vi "Kinesis - KBD101 - Set Trigger Parameters.vi"() -> ()   [LabVIEW 2012]
uses:
  U:/Kinesis LabVIEW Website Examples/Thorlabs.MotionControl.Controls.dll
  Thorlabs.MotionControl.Controls.dll
  U:/Kinesis LabVIEW Website Examples/Thorlabs.MotionControl.KCube.BrushlessMotorCLI.dll
  Thorlabs.MotionControl.KCube.BrushlessMotorCLI.dll
  U:/Kinesis LabVIEW Website Examples/Thorlabs.MotionControl.GenericMotorCLI.dll
  Thorlabs.MotionControl.GenericMotorCLI.dll
panel:
  in  "?":bool
  in  "stop":bool
  in  "SerialNumber":string
  in  "Trigger2Polarity":i32(ring)=1 items=["TriggerHigh"=1, "TriggerLow"=2]
  in  "Trigger2Mode":i32(ring) items=["Disabled"=0, "TrigIN_GPI"=1, "TrigIN_RelativeMove"=2, "TrigIN_AbsoluteMove"=3, "TrigIN_KCubeTriggerParams"=4, "TrigOUT_GPO"=10, "TrigOUT_InMotion"=11, "TrigOUT_AtMaxVelocity"=12, "TrigOUT_AtPositionFwd"=13, "TrigOUT_AtPositionRev"=14, "TrigOUT_AtPositionBoth"=15, "TrigOut_AtFwdLimit"=16, "TrigOut_AtBwdLimit"=17, "TrigOut_AtLimit"=18]
  in  "Trigger1Polarity":i32(ring)=1 items=["TriggerHigh"=1, "TriggerLow"=2]
  out "Trigger2Polarity":i32(ring)=1 items=["TriggerHigh"=1, "TriggerLow"=2]
  out "Trigger2Mode":i32(ring) items=["Disabled"=0, "TrigIN_GPI"=1, "TrigIN_RelativeMove"=2, "TrigIN_AbsoluteMove"=3, "TrigIN_KCubeTriggerParams"=4, "TrigOUT_GPO"=10, "TrigOUT_InMotion"=11, "TrigOUT_AtMaxVelocity"=12, "TrigOUT_AtPositionFwd"=13, "TrigOUT_AtPositionRev"=14, "TrigOUT_AtPositionBoth"=15, "TrigOut_AtFwdLimit"=16, "TrigOut_AtBwdLimit"=17, "TrigOut_AtLimit"=18]
  out "Trigger1Polarity":i32(ring)=1 items=["TriggerHigh"=1, "TriggerLow"=2]
  in  "Trigger1Mode":i32(ring) items=["Disabled"=0, "TrigIN_GPI"=1, "TrigIN_RelativeMove"=2, "TrigIN_AbsoluteMove"=3, "TrigIN_KCubeTriggerParams"=4, "TrigOUT_GPO"=10, "TrigOUT_InMotion"=11, "TrigOUT_AtMaxVelocity"=12, "TrigOUT_AtPositionFwd"=13, "TrigOUT_AtPositionRev"=14, "TrigOUT_AtPositionBoth"=15, "TrigOut_AtFwdLimit"=16, "TrigOut_AtBwdLimit"=17, "TrigOut_AtLimit"=18]
  out "Trigger1Mode":i32(ring) items=["Disabled"=0, "TrigIN_GPI"=1, "TrigIN_RelativeMove"=2, "TrigIN_AbsoluteMove"=3, "TrigIN_KCubeTriggerParams"=4, "TrigOUT_GPO"=10, "TrigOUT_InMotion"=11, "TrigOUT_AtMaxVelocity"=12, "TrigOUT_AtPositionFwd"=13, "TrigOUT_AtPositionRev"=14, "TrigOUT_AtPositionBoth"=15, "TrigOut_AtFwdLimit"=16, "TrigOut_AtBwdLimit"=17, "TrigOut_AtLimit"=18]
  in  "TriggerStartPositionRev":dbl
  in  "TriggerStartPositionFwd":dbl
  in  "TriggerPulseWidth":i32
  in  "TriggerIntervalRev":dbl
  in  "TriggerIntervalFwd":dbl
  in  "TriggerCountRev":i32
  in  "CycleCount":i32
  in  "TriggerCountFwd":i32
  out "TriggerStartPositionRev":dbl
  out "TriggerStartPositionFwd":dbl
  out "TriggerPulseWidth":i32
  out "TriggerIntervalRev":dbl
  out "TriggerIntervalFwd":dbl
  out "TriggerCountRev":i32
  out "TriggerCountFwd":i32
  out "CycleCount":i32
  in  "KCubeBrushlessControl":refnum<k24>(container)
  # "Notes:"
  # "- Ensure that the appropriate .DLLs are copied into your Project Folder. Check that the correct bit type are used depending on your version of LabVIEW\ni.e. 32-bit or 64-bit.\n\n\n\n\n\n\n\n\n\n\n\n\n\n\n- Open the example VI through the LabVIEW Project Explorer to correctly load the User Interface from Thorlabs.MotionControl.Controls.dll."
  # "Thorlabs Hardware: KBD101 - K-Cube Brushless DC Servo Motor Controller\nhttps://www.thorlabs.com/thorproduct.cfm?partnumber=KBD101\n\nDescription: This VI will enable you to explore the Trigger Parameters available to all Thorlabs K-Cube devices. In this case, the VI will accept a KBD101 controller specifically.\n\nInstructions: \n1) Connect your KBD101 device to your PC & power the device, ensuring your stage/actutator is connected. For full device setup, the device product manual can be found on our website here. - https://www.thorlabs.com/thorproduct.cfm?partnumber=KBD101\n2) Enter the device serial number below.\n3) Click 'Run' in the LabVIEW Toolbar.\n4) Enter parameters for Trigger Settings in the controls below. Further details of these parameters are outlined in the KBD101 product manual, as well as the Kinesis .NET API.\n5) Click 'SET TRIG PARAMETERS' to set the Trigger Parameters. The program will poll for clicks every 500ms.\n6) Click 'END PROGRAM' to end the VI."
  # "Example Image of .NET Controller - VI opened via Project Explorer/ not opened via Project Explorer"
  # "VI Not Opened via Project Explorer"
  # "VI Opened via Project Explorer"
  # "- To explore the range of methods available, please visit the .NET API, included with your Kinesis software.\n\n- For tips on building your own VIs with Thorlabs Motion Control Hardware, please see our LabVIEW Guide here.\nhttps://www.thorlabs.com/newgrouppage9.cfm?objectgroup_id=10285"
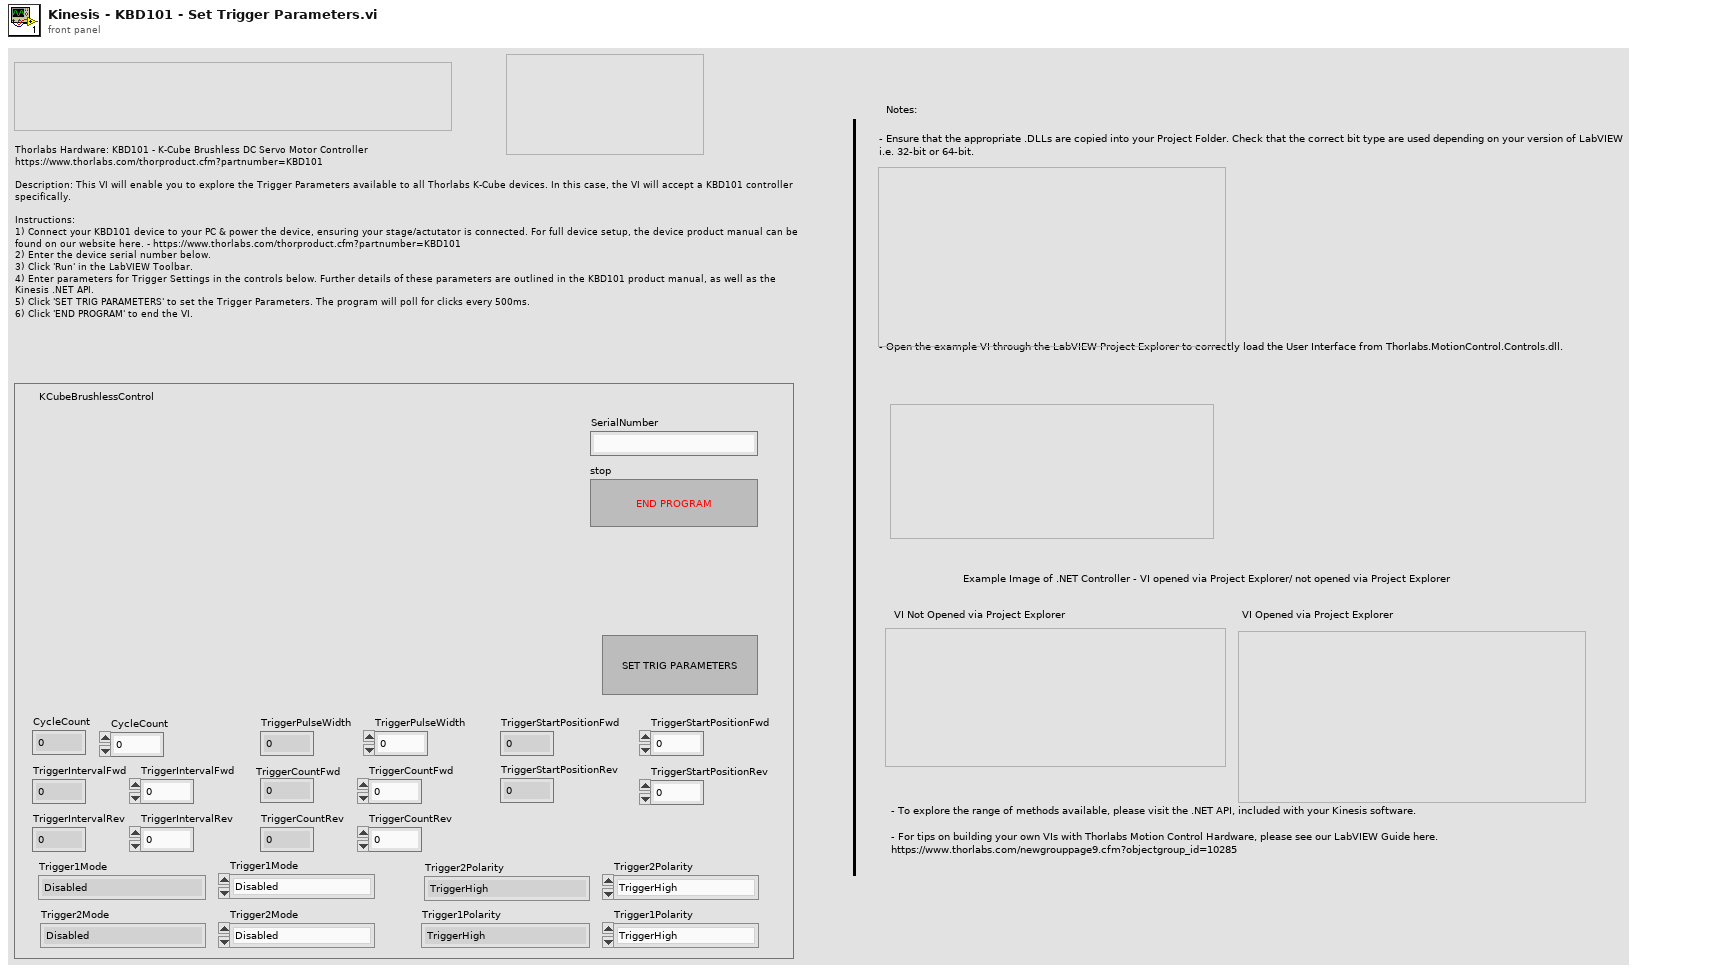
[diagram p1: front panel]
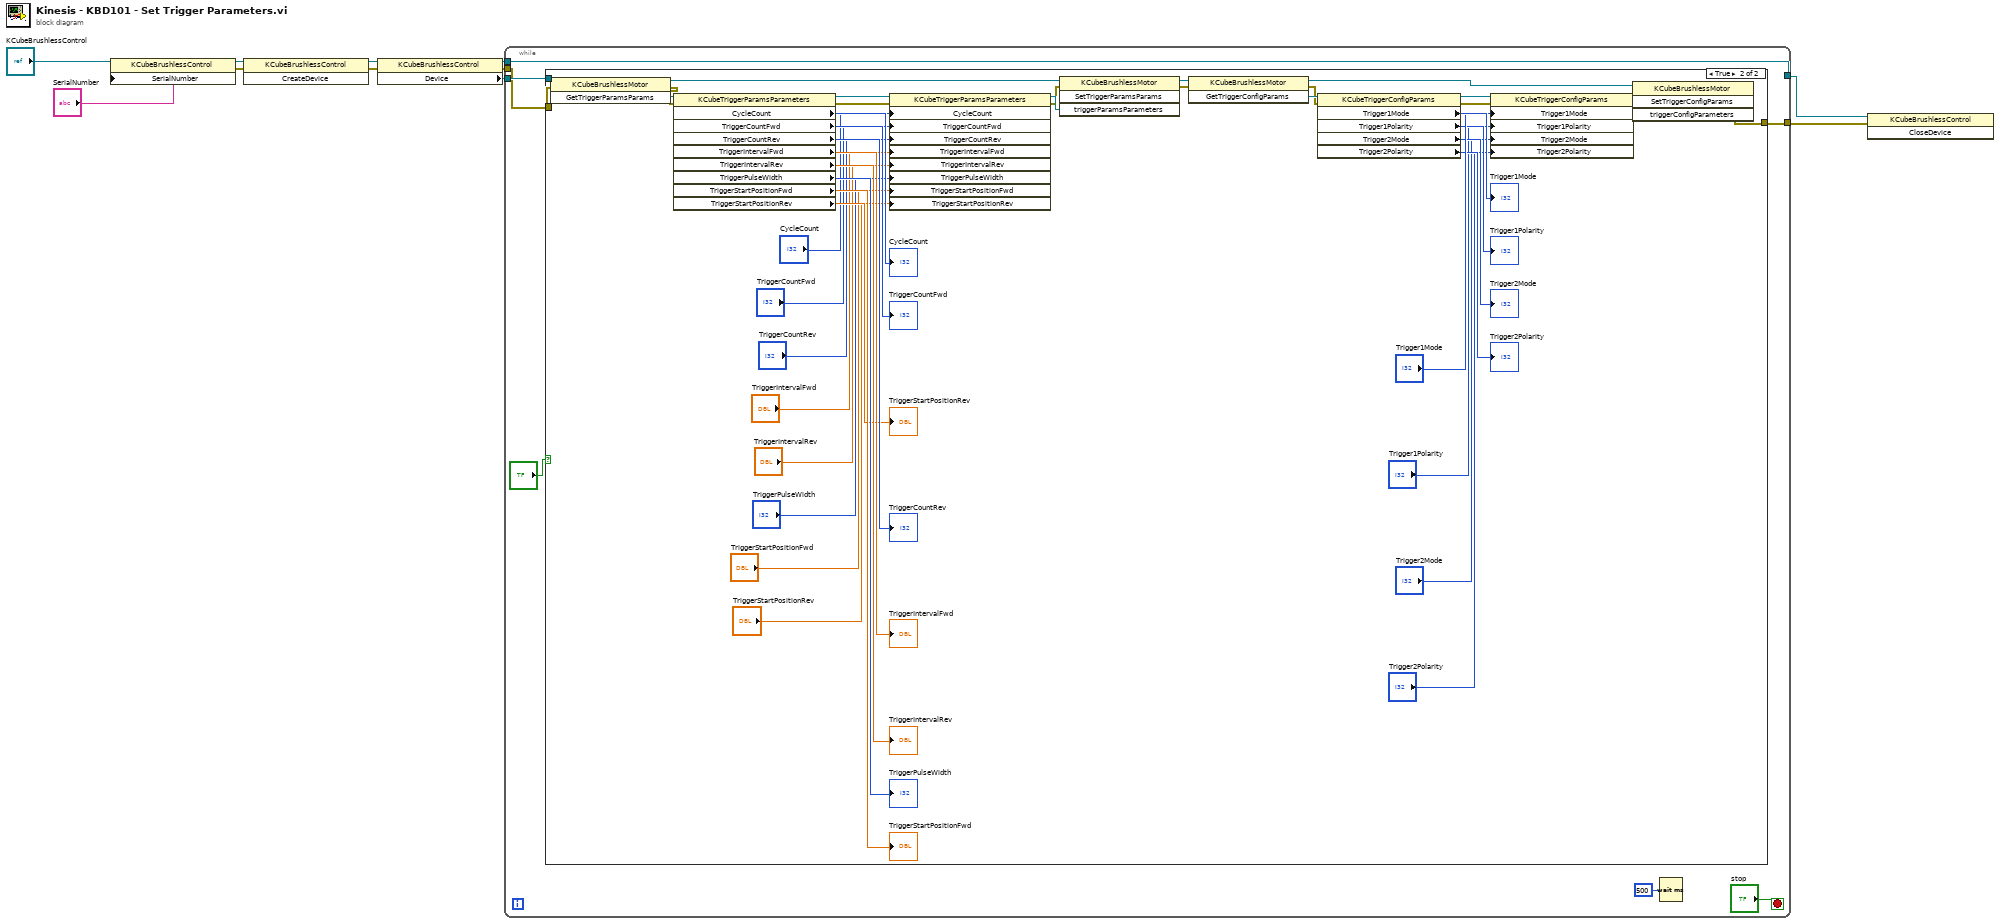
[diagram p0: block diagram]
diagram:
  n1 = property class="KCubeBrushlessControl"(reference="KCubeBrushlessControl", "SerialNumber"="SerialNumber") -> (reference out=w10:refnum<k24>, error out=w4:errorcluster)  [unwired: 1 in]
  n2 = invoke class="KCubeBrushlessControl" method="CreateDevice"(reference=w10, error in=w4) -> (reference out=w9:refnum<k24>, error out=w3:errorcluster)  [unwired: 1 in, 1 out]
  n3 = property class="KCubeBrushlessControl"(reference=w9, error in=w3) -> (reference out=w6:refnum<k24>, error out=w2:errorcluster, "Device"=w8:refnum<k24>)
  n4 = while {
    tunnel: w8 -> [w18]
    tunnel: [w16] -> w5
    tunnel: w6 -> [w16]
    tunnel: w2 -> [w15]
    tunnel: [w14] -> w1
    stop <- "stop" stop-if-true
    n5 = case shown="True" "?" {
      tunnel: w18 -> [_ w62]
      tunnel: w15 -> [w19 w28]
      tunnel: [w19 w20] -> w14
      frame False {
      }
      frame True {
        n6 = invoke class="KCubeBrushlessMotor" method="GetTriggerParamsParams"(reference=w62, error in=w28) -> (reference out=w60:refnum<k24>, error out=w27:errorcluster, "GetTriggerParamsParams"=w61:refnum<k24>)  [unwired: 1 in]
        n7 = property class="KCubeTriggerParamsParameters"(reference=w61, error in=w27) -> (reference out=w59:refnum<k24>, error out=w26:errorcluster, "CycleCount"=→"CycleCount":i32, "TriggerCountFwd"=→"TriggerCountFwd":i32, "TriggerCountRev"=→"TriggerCountRev":i32, "TriggerIntervalFwd"=→"TriggerIntervalFwd":dbl, "TriggerIntervalRev"=→"TriggerIntervalRev":dbl, "TriggerPulseWidth"=→"TriggerPulseWidth":i32, "TriggerStartPositionFwd"=→"TriggerStartPositionFwd":dbl, "TriggerStartPositionRev"=→"TriggerStartPositionRev":dbl)
        n8 = property class="KCubeTriggerParamsParameters"(reference=w59, error in=w26, "CycleCount"="CycleCount", "TriggerCountFwd"="TriggerCountFwd", "TriggerCountRev"="TriggerCountRev", "TriggerIntervalFwd"="TriggerIntervalFwd", "TriggerIntervalRev"="TriggerIntervalRev", "TriggerPulseWidth"="TriggerPulseWidth", "TriggerStartPositionFwd"="TriggerStartPositionFwd", "TriggerStartPositionRev"="TriggerStartPositionRev") -> (reference out=w58:refnum<k24>, error out=w25:errorcluster)
        n9 = invoke class="KCubeBrushlessMotor" method="SetTriggerParamsParams"(reference=w60, error in=w25, "triggerParamsParameters"=w58) -> (reference out=w57:refnum<k24>, error out=w24:errorcluster)  [unwired: 1 in, 2 out]
        n10 = invoke class="KCubeBrushlessMotor" method="GetTriggerConfigParams"(reference=w57, error in=w24) -> (reference out=w53:refnum<k24>, error out=w23:errorcluster, "GetTriggerConfigParams"=w56:refnum<k24>)  [unwired: 1 in]
        n11 = property class="KCubeTriggerConfigParams"(reference=w56, error in=w23) -> (reference out=w55:refnum<k24>, error out=w22:errorcluster, "Trigger1Mode"=→"Trigger1Mode":i32, "Trigger1Polarity"=→"Trigger1Polarity":i32, "Trigger2Mode"=→"Trigger2Mode":i32, "Trigger2Polarity"=→"Trigger2Polarity":i32)
        n12 = property class="KCubeTriggerConfigParams"(reference=w55, error in=w22, "Trigger1Mode"="Trigger1Mode", "Trigger1Polarity"="Trigger1Polarity", "Trigger2Mode"="Trigger2Mode", "Trigger2Polarity"="Trigger2Polarity") -> (reference out=w54:refnum<k24>, error out=w21:errorcluster)
        n13 = invoke class="KCubeBrushlessMotor" method="SetTriggerConfigParams"(reference=w53, error in=w21, "triggerConfigParameters"=w54) -> (error out=w20:errorcluster)  [unwired: 1 in, 3 out]
      }
    }
    n14 = Wait (ms)(milliseconds to wait=u32 500) -> ()  [unwired: 1 out]
  }
  n15 = invoke class="KCubeBrushlessControl" method="CloseDevice"(reference=w5, error in=w1) -> ()  [unwired: 1 in, 3 out]
